vi "Program list Selection.vi"() -> (1 "Exit":bool, 2 "String":string)   [LabVIEW 2015]
uses:
  Control Button/Exit.ctl
  Control Button/next.ctl
  Galobal variable_TI.vi
panel:
  out "String 2":string
  in  "Next":T1
  in  "Exit":T2
  in  "Program List":string(combo)
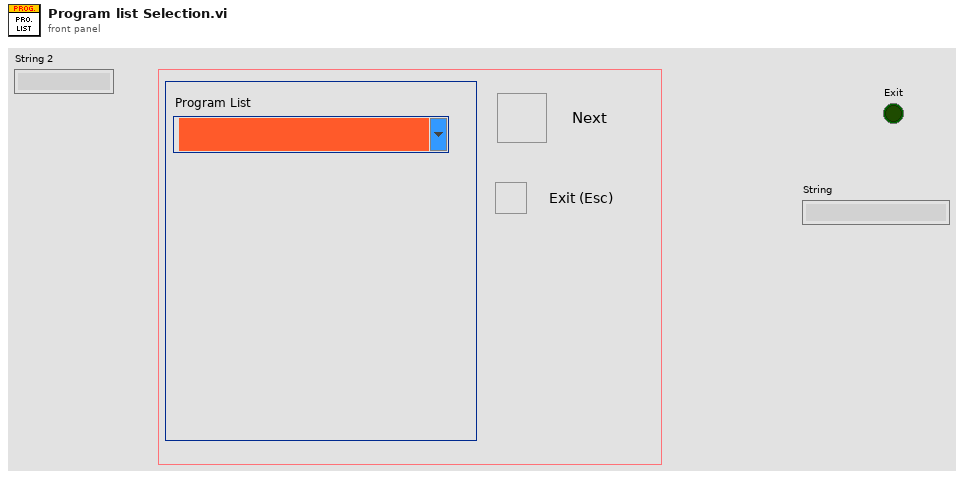
[diagram p1: front panel]
types:
  T1 = typedef "next.ctl" = bool
  T2 = typedef "Exit.ctl" = bool
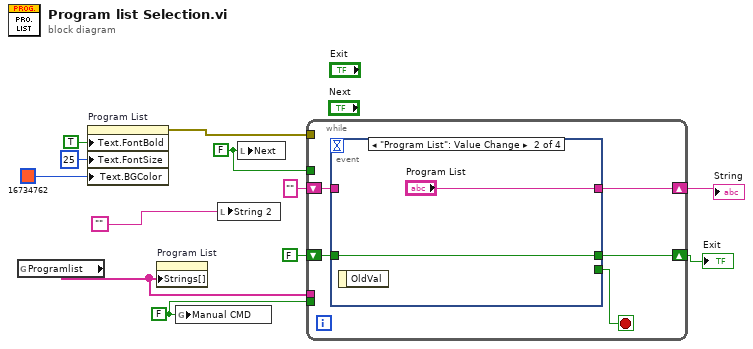
[diagram p0: block diagram]
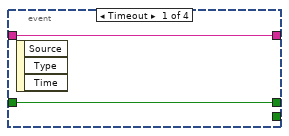
[diagram p2: hidden frame]
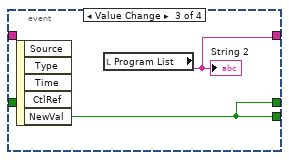
[diagram p3: hidden frame]
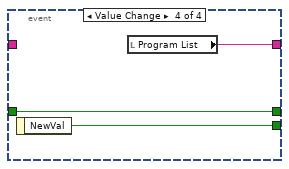
[diagram p4: hidden frame]
diagram:
  w1 = FALSE ("Manual CMD")
  w2 = FALSE ("Next")
  n1 = global read "Galobal variable_TI.vi" "Programlist"() -> (w8:string[])
  n2 = property on="Program List" class="CmbBox"("Text.FontBold"=TRUE ("Text.Font:Bold"), "Text.FontSize"=u32 25 ("Text.Font:Size"), "Text.BGColor"=u32 16734762 ("Color Box")) -> (error out=w5:errorcluster)  [unwired: 2 in, 1 out]
  n3 = property on="Program List" class="CmbBox"("Strings[]"=w8) -> ()  [unwired: 2 in, 2 out]
  n4 = global write "Galobal variable_TI.vi" "Manual CMD"(w1) -> ()
  n5 = local write "String 2"("") -> ()
  n6 = local write "Next"(w2) -> ()
  n7 = while {
    shift-right: [w17] -> w12
    shift-left: "" ("Combo Box") -> [w16]
    shift-right: [w14] -> w9
    shift-left: T2 FALSE ("NewVal") -> [w13]
    tunnel: w8 -> [_]
    tunnel: w5 -> [_]
    tunnel: w2 -> [_]
    tunnel: w1 -> [_]
    stop <- w15 stop-if-true
    n8 = event shown="[1] \"Program List\": Value Change" {
      selector: _ -> [_ _ _ _]
      dyn-events: _ -> [_ _ _ _]
      timeout: _ -> [_ _ _ _]
      tunnel: [w19 "Program List" w23 w25] -> w17
      tunnel: w16 -> [w19 _ _ _]
      tunnel: [_ _ w22 w26] -> w15
      tunnel: [w18 w20 w22 w24] -> w14
      tunnel: w13 -> [w18 w20 _ w24]
      event Timeout {
        n9 = event-data() -> ()  [unwired: 1 in, 3 out]
      }
      event "Program List": Value Change {
        n10 = event-data() -> ()  [unwired: 1 in, 1 out]
      }
      event Value Change {
        n11 = event-data() -> ("NewVal"=w22:T1)  [unwired: 1 in, 4 out]
        n12 = local read "Program List"() -> (w23:string)
        "String 2" <- w23
      }
      event Value Change {
        n13 = event-data() -> ("NewVal"=w26:T2)  [unwired: 1 in]
        n14 = local read "Program List"() -> (w25:string)
      }
    }
  }
  "String" <- w12
  "Exit" <- w9
